vi "Shutdown.vi"(8 "error in (no error)":errorcluster, 11 "Renderer":refnum<class "Renderer.lvclass">) -> (0 "error out":errorcluster)   [LabVIEW 2021, in "Renderer.lvclass"]
uses:
  Renderer.lvclass
  Renderer.lvclass/Renderer.ctl
  LabSDL2/Source/Libraries/LibSDL2 Wrapper/LibSDL2.lvlib
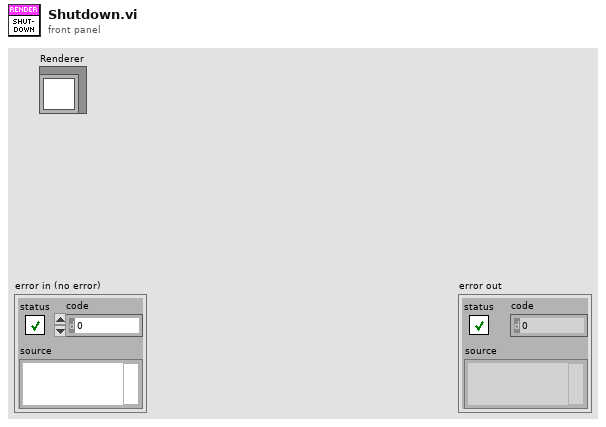
[diagram p1: front panel]
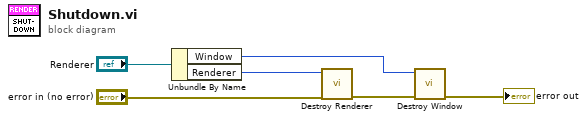
[diagram p0: block diagram]
diagram:
  n1 = Unbundle By Name("Renderer") -> ("Window"=w6:u32, "Renderer"=w4:u32)
  n2 = call "Destroy Renderer.vi"("error in"="error in (no error)", "Renderer Pointer"=w4) -> ("error out"=w5:errorcluster)  [unwired: 9 in]
  n3 = call "Destroy Window.vi"("error in"=w5, "Window Pointer"=w6) -> ("error out"=→"error out":errorcluster)  [unwired: 9 in]
